vi "image_to_bits.vi"(3 "Packet\nMessage Length (bits)":i32, 5 "path to JPEG file":path) -> (0 "Number of Packets":i32, 1 "message bitstream":i8[](array[numeric]), 2 "Transmitted picture":picture)   [LabVIEW 2019]
uses:
  <vilib>/picture/picture.llb/Draw True-Color Pixmap.vi
panel:
  out "Array":i8[][](array[numeric])
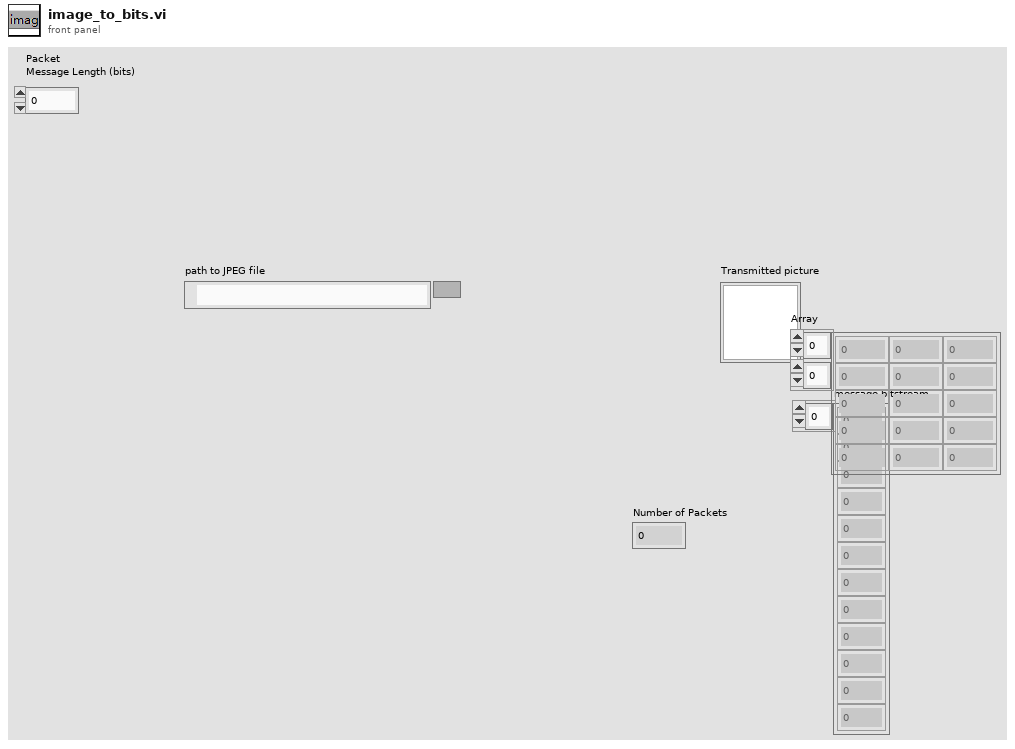
[diagram p1: front panel]
types:
  T1 = typedef "imagedata.ctl" = cluster{"image type":i32, "image depth":i32, "image":u8[], "mask":u8[], "colors":u32[], "Rectangle":cluster{"left":i16, "top":i16, "right":i16, "bottom":i16}}
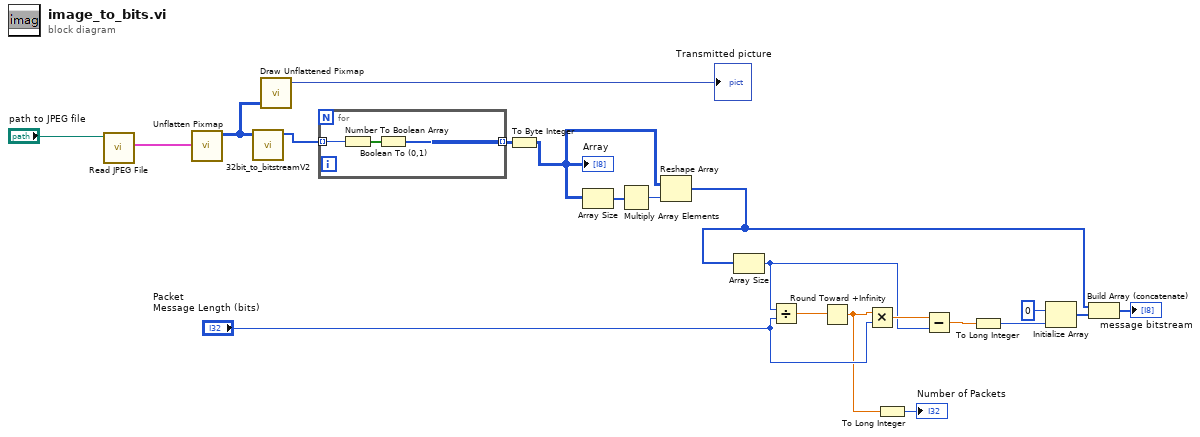
[diagram p0: block diagram]
diagram:
  n1 = call <vilib>:"Read JPEG File.vi"("path to JPEG file"="path to JPEG file") -> ("image data"=w20:T1)  [unwired: 8 in, 2 out]
  n2 = call <vilib>:"Unflatten Pixmap.vi"("image data"=w20) -> ("24-bit pixmap"=w19:u32[][])  [unwired: 4 in, 6 out]
  n3 = call "32bit_to_bitstreamV2.vi"("24-bit pixmap"=w19) -> ("Bitstream with Guard"=w6:u8[])  [unwired: 7 in, 1 out]
  n4 = call-poly <vilib>:"Draw Unflattened Pixmap.vi"("data (RGB format)"=w19) -> ("new picture"=→"Transmitted picture":picture)  [unwired: 8 in]
  n5 = for {
    tunnel: w6 -> [w24] mode=indexing
    tunnel: [w22] -> w5 mode=indexing
    n6 = Number To Boolean Array(number=w24) -> (Boolean array=w23:bool[])
    n7 = Boolean To (0,1)(Boolean=w23) -> (0, 1=w22:i16[])
  }
  n8 = To Byte Integer(number=w5) -> (8bit integer=w2:i8[][])
  "Array" <- w2
  n9 = Array Size(array=w2) -> (size(s)=w4:i32[])
  n10 = Multiply Array Elements(1:w4) -> (0:w3:i32)
  n11 = Reshape Array "Reshape Array"(w2, w3) -> (w1:i8[])
  n12 = Array Size(array=w1) -> (size(s)=w14:i32)
  n13 = Divide(x=w14, y="Packet\nMessage Length (bits)") -> (x/y=w17:dbl)
  n14 = Round Toward +Infinity(x=w17) -> (ceil(x): smallest int >= x=w7:dbl)
  n15 = Multiply(x=w7, y="Packet\nMessage Length (bits)") -> (x*y=w15:dbl)
  n16 = To Long Integer(number=w7) -> (32bit integer=→"Number of Packets":i32)
  n17 = Subtract(x=w15, y=w14) -> (x-y=w9:dbl)
  n18 = To Long Integer(number=w9) -> (32bit integer=w12:i32)
  n19 = Initialize Array "Initialize Array"(i8 0 ("element"), w12) -> (w11:i8[])
  n20 = Build Array (concatenate) "Build Array"(w1, w11) -> (→"message bitstream":i8[])
